vi "array_decimate_test.vi"() -> ()   [LabVIEW 2010]
panel:
  out "Array 2":dbl[][](array[numeric])
  in  "Array":dbl[](array[numeric])
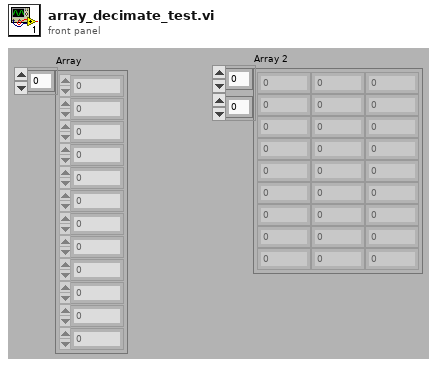
[diagram p1: front panel]
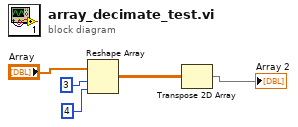
[diagram p0: block diagram]
diagram:
  n1 = Reshape Array("Array", 3, 4) -> (w5:dbl[][])
  n2 = Transpose 2D Array(2D array=w5) -> (transposed array=→"Array 2":dbl[][])
